vi "ECGfirst.vi"() -> ()   [LabVIEW 2015]
uses:
  <vilib>/Instr/_visa.llb/VISA Configure Serial Port (Instr).vi
panel:
  in  "Stop Button 2":bool
  in  "Menus":enum32{"Configuración", "Variables", "Graficas"}(tab)
  out "A case":u16
  in  "Text & Pict Ring 2":u16(ring) items=["Tiempo Real"=1, "Desconectado"=2, "Datos almaceados"=3, "Alarma Medir"=0]
  in  "LECTURA":bool
  in  "ESCRITURA":bool
  in  "VISA resource name":refnum<visa-resource-name>
  out "Al PIC":string
  out "Array 2":dbl[](array[numeric])
  out "read buffer":string
  out "Table":string[][](table)
  in  "Open Button":bool
  out "Table Control":string[][](table)
  in  "path":path
  out "Waveform Chart":dbl(graph)
  # "ELECTROCARDIOGRAFO \nPORTATIL"
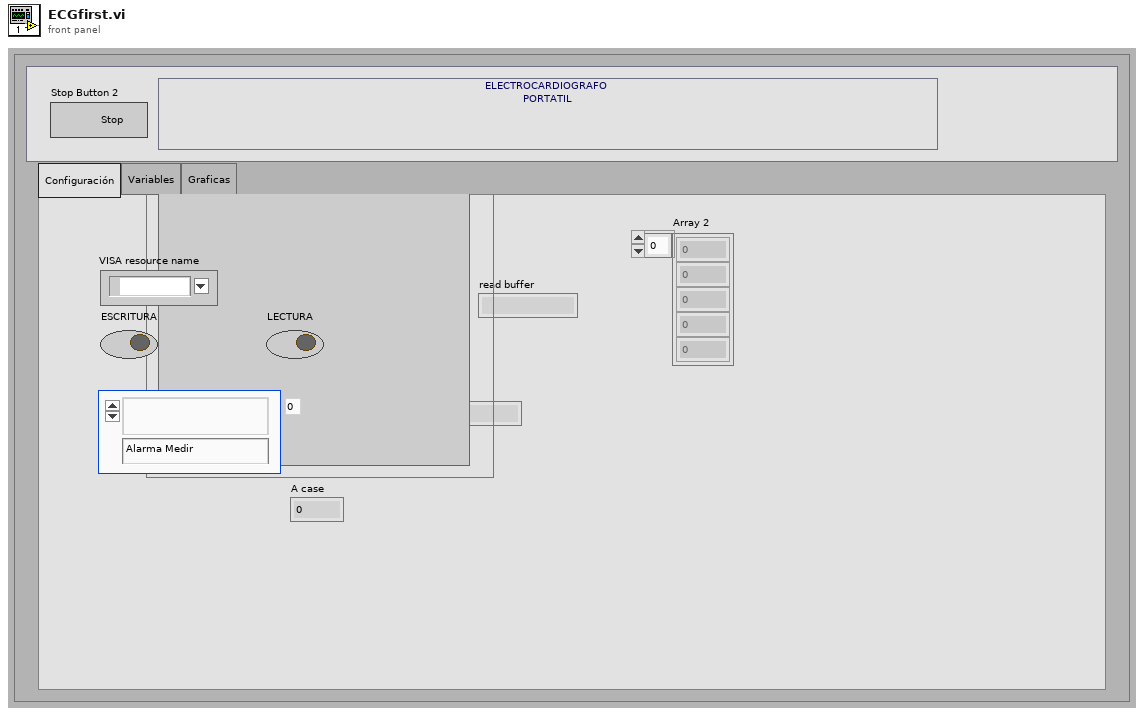
[diagram p1: front panel]
types:
  T1 = cluster{"Excel._Application":refnum<k7>, "Workbooks":refnum<k7>}
  T2 = cluster{"Excel._Application":refnum<k7>, "Workbooks":refnum<k7>, "Open":refnum<k7>}
  T3 = cluster{"Excel._Application":refnum<k7>, "Workbooks":refnum<k7>, "Open":refnum<k7>, "Worksheets":refnum<k7>, "Excel._Worksheet":refnum<k7>}
  T4 = cluster{"unsigned byte array[0]":u8, "unsigned byte array[1]":u8, "unsigned byte array[2]":u8, "unsigned byte array[3]":u8, "unsigned byte array[4]":u8, "unsigned byte array[5]":u8, "unsigned byte array[6]":u8, "unsigned byte array[7]":u8, "unsigned byte array[8]":u8}
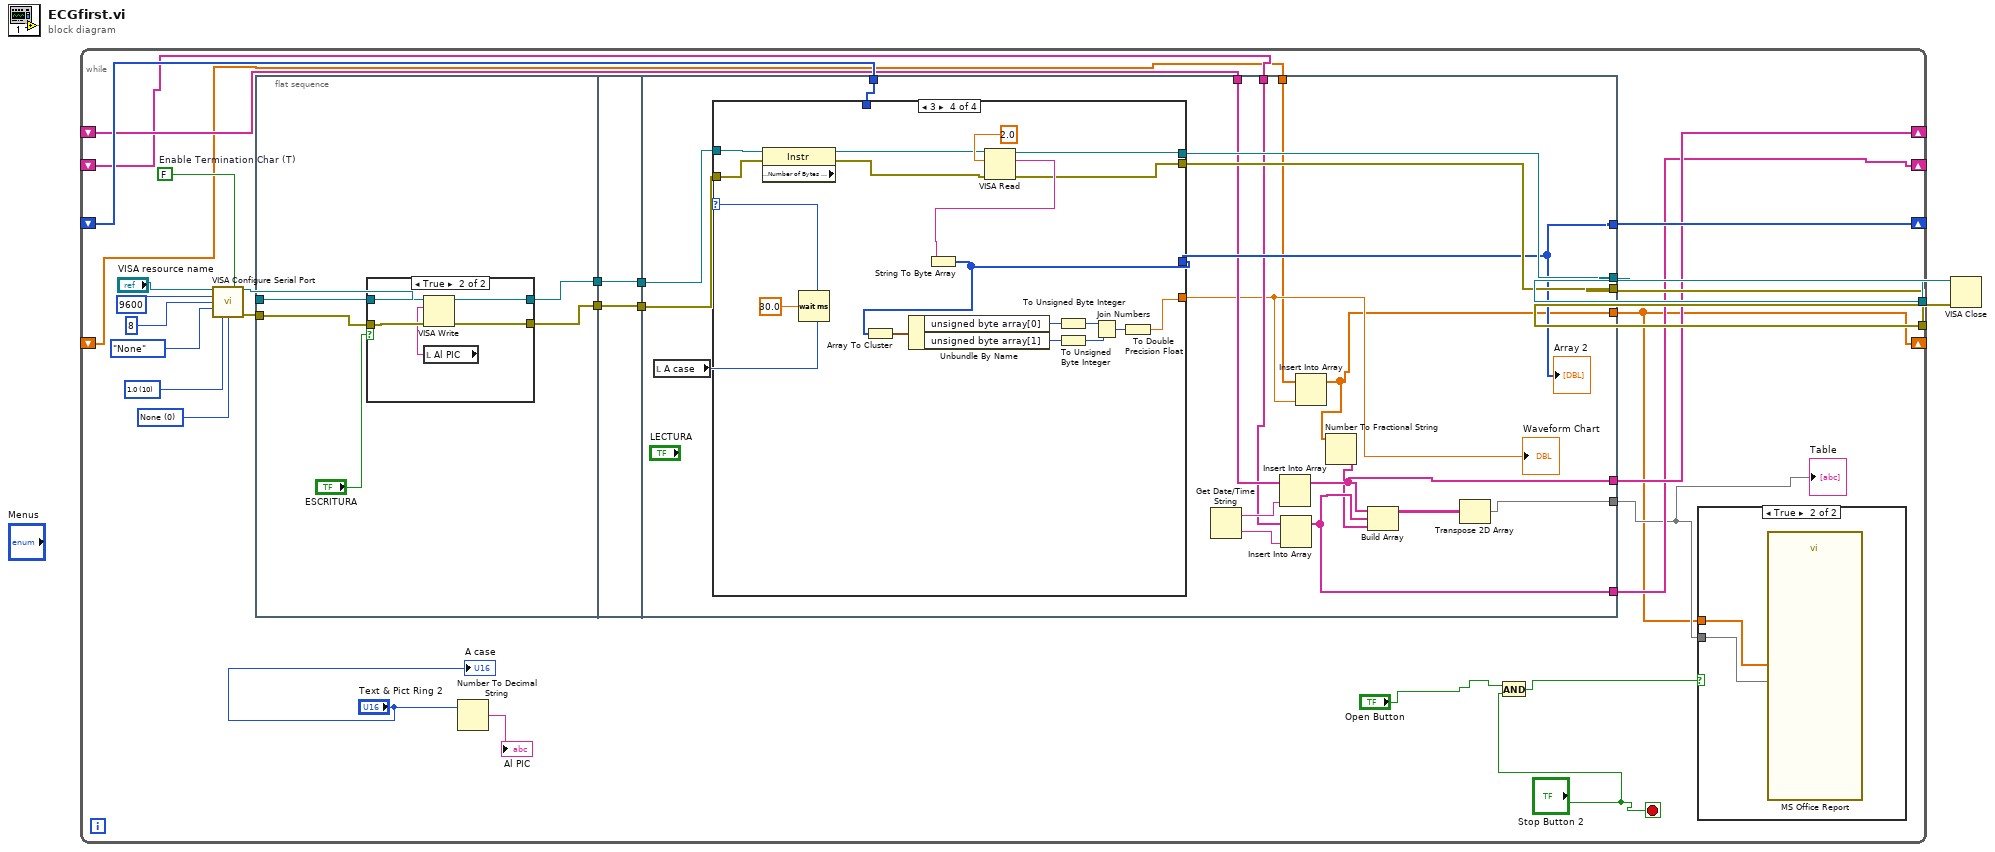
[diagram p0: block diagram]
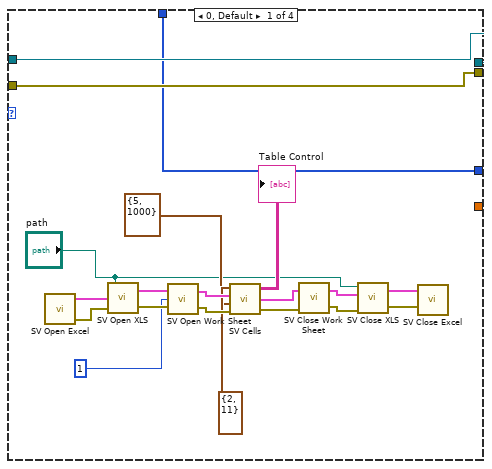
[diagram p4: hidden frame]
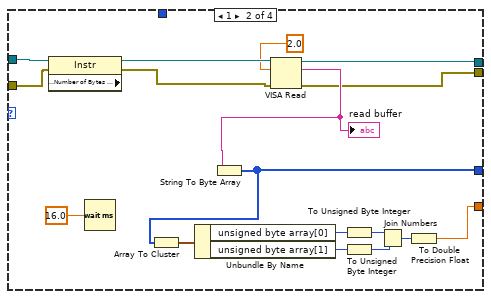
[diagram p5: hidden frame]
diagram:
  n1 = while {
    tunnel: [w17] -> w2
    tunnel: [w15] -> w1
    shift-right: [w14] -> _
    shift-left: _ -> [w13]
    shift-right: [w12] -> _
    shift-left: _ -> [w11]
    shift-right: [w10] -> _
    shift-left: _ -> [w9]
    shift-right: [w3] -> _
    shift-left: _ -> [w4]
    stop <- "Stop Button 2" stop-if-true
    w31 = u16 0 items=["None", "XON/XOFF", "RTS/CTS", "XON/XOFF & RTS/CTS", "DTR/DSR", "XON/XOFF & DTR/DSR"] ("flow control (0:none)")
    w30 = FALSE  # Enable Termination Char (T)
    w27 = u16 10 items=["1.0"=10, "1.5"=15, "2.0"=20] ("stop bits (10: 1 bit)")
    n2 = call-poly "VISA Configure Serial Port"("VISA resource name"="VISA resource name", "Enable Termination\nChar (T)"=w30, "baud rate (9600)"=9600 ("Numeric 2"), "data bits (8)"=u16 8, "parity (0:none)"=enum16{"None", "Odd", "Even", "Mark", "Space"}."None", "stop bits (10: 1 bit)"=w27, "flow control (0:none)"=w31) -> ("VISA resource name out"=w19:refnum<visa-resource-name>, "error out"=w18:errorcluster)  [unwired: 7 in]
    n3 = flat-sequence {
      tunnel: [w35] -> w23
      tunnel: [w34] -> w22
      tunnel: w19 -> [w38]
      tunnel: w18 -> [w37]
      tunnel: [w47] -> w21
      tunnel: w23 -> [w47]
      tunnel: w22 -> [w46]
      tunnel: [w46] -> w20
      tunnel: w21 -> [w65]
      tunnel: w20 -> [w64]
      tunnel: [w63] -> w17
      tunnel: [w62] -> w15
      tunnel: [w61] -> w14
      tunnel: w13 -> [w60]
      tunnel: [w57] -> w12
      tunnel: w11 -> [w56]
      tunnel: [w55] -> w10
      tunnel: w9 -> [w54]
      tunnel: [w52] -> w8
      tunnel: [w48] -> w3
      tunnel: w4 -> [w50]
      frame #0 {
        n4 = case shown="True" "ESCRITURA" {
          tunnel: w38 -> [w40 w45]
          tunnel: [w40 w41] -> w35
          tunnel: [w39 w44] -> w34
          tunnel: w37 -> [w39 w43]
          frame False {
          }
          frame True {
            n5 = local read "Al PIC"() -> (w42:string)
            n6 = VISA Write(VISA resource name=w45, write buffer=w42, error in (no error)=w43) -> (VISA resource name out=w41:refnum<visa-resource-name>, error out=w44:errorcluster)  [unwired: 1 out]
          }
        }
      }
      frame #1 {
      }
      frame #2 {
        n7 = local read "A case"() -> (w66:u16)
        n8 = case shown="3" w66 {
          tunnel: w65 -> [w86 w92 w106 w112]
          tunnel: w64 -> [w85 w91 w105 w111]
          tunnel: [w86 w90 w106 w110] -> w63
          tunnel: [w85 w89 w105 w109] -> w62
          tunnel: [_ w88 _ w107] -> w51
          tunnel: [w84 w87 w104 w108] -> w61
          tunnel: w60 -> [w84 _ w104 _]
          frame 0, Default {
            n9 = call "SV Open Excel.vi"() -> ("error out"=w83:errorcluster, "Refnum Cluster"=w82:T1)  [unwired: 1 in]
            n10 = call "SV Open XLS.vi"("error in"=w83, "Refnum Cluster In"=w82, "path"="path") -> ("error out"=w80:errorcluster, "Refnum Cluster Out"=w81:T2)
            n11 = call "SV Open Work Sheet.vi"("error in (no error)"=w80, "Sheet"=1, "Refnum Cluster In"=w81) -> ("error out"=w78:errorcluster, "Refnum Cluster Out"=w79:T3)
            n12 = call "SV Cells.vi"("error in"=w78, "End 2"=cluster{"Column":i32, "Row":i32} {"Column"=5, "Row"=1000}, "Refnum Cluster In"=w79, "Start 2"=cluster{"Column":i32, "Row":i32} {"Column"=2, "Row"=11}) -> ("Error Out"=w77:errorcluster, "Refnum Cluster Out"=w76:T3, "Data"=→"Table Control":string[][])
            n13 = call "SV Close Work Sheet.vi"("error in (no error)"=w77, "Refnum Cluster In"=w76) -> ("error out"=w74:errorcluster, "Refnum Cluster Out"=w75:T2)
            n14 = call "SV Close XLS.vi"("error in (no error)"=w74, "Refnum Cluster In"=w75, "path 2"="path") -> ("error out"=w72:errorcluster, "Refnum Cluster Out"=w73:T1)  [unwired: 1 in]
            n15 = call "SV Close Excel.vi"("error in (no error)"=w72, "Refnum Cluster In"=w73) -> ()  [unwired: 1 out]
          }
          frame 1 {
            n16 = property class="Instr" props=["Serial Settings:Number of Bytes at Serial Port"](reference=w92, error in=w91) -> (reference out=w101:refnum<visa-resource-name>, error out=w102:errorcluster)  [unwired: 1 out]
            n17 = Wait (ms)(milliseconds to wait=sgl 16.0 ("Vielfache von ms")) -> ()  [unwired: 1 out]
            n18 = VISA Read(VISA resource name=w101, byte count=2.0 ("BYTES A LEER"), error in (no error)=w102) -> (VISA resource name out=w90:refnum<visa-resource-name>, read buffer=w93:string, error out=w89:errorcluster)  [unwired: 1 out]
            "read buffer" <- w93
            n19 = String To Byte Array(string=w93) -> (unsigned byte array=w87:u8[])
            n20 = Array To Cluster(array=w87) -> (cluster=w94:T4)
            n21 = Unbundle By Name(w94) -> ("unsigned byte array[0]"=w98:u8, "unsigned byte array[1]"=w99:u8)
            n22 = To Unsigned Byte Integer(number=w98) -> (unsigned 8bit integer=w95:u8)
            n23 = To Unsigned Byte Integer(number=w99) -> (unsigned 8bit integer=w96:u8)
            n24 = Join Numbers(hi=w95, lo=w96) -> ((hi.lo)=w97:u16)
            n25 = To Double Precision Float(number=w97) -> (double precision float=w88:dbl)
          }
          frame 2 {
          }
          frame 3 {
            n26 = property class="Instr" props=["Serial Settings:Number of Bytes at Serial Port"](reference=w112, error in=w111) -> (reference out=w115:refnum<visa-resource-name>, error out=w114:errorcluster)  [unwired: 1 out]
            n27 = Wait (ms)(milliseconds to wait=sgl 30.0 ("Vielfache von ms")) -> ()  [unwired: 1 out]
            n28 = VISA Read(VISA resource name=w115, byte count=2.0 ("BYTES A LEER"), error in (no error)=w114) -> (VISA resource name out=w110:refnum<visa-resource-name>, read buffer=w123:string, error out=w109:errorcluster)  [unwired: 1 out]
            n29 = String To Byte Array(string=w123) -> (unsigned byte array=w108:u8[])
            n30 = Array To Cluster(array=w108) -> (cluster=w122:T4)
            n31 = Unbundle By Name(w122) -> ("unsigned byte array[0]"=w118:u8, "unsigned byte array[1]"=w117:u8)
            n32 = To Unsigned Byte Integer(number=w118) -> (unsigned 8bit integer=w121:u8)
            n33 = To Unsigned Byte Integer(number=w117) -> (unsigned 8bit integer=w120:u8)
            n34 = Join Numbers(hi=w121, lo=w120) -> ((hi.lo)=w119:u16)
            n35 = To Double Precision Float(number=w119) -> (double precision float=w107:dbl)
          }
        }
        "Waveform Chart" <- w51
        "Array 2" <- w61
        n36 = Get Date/Time String() -> (date string=w59:string, time string=w58:string)  [unwired: 3 in]
        n37 = Insert Into Array(array=w56, new element=w59) -> (w57:string[])  [unwired: 1 in]
        n38 = Insert Into Array(array=w54, new element=w58) -> (w55:string[])  [unwired: 1 in]
        n39 = Insert Into Array(array=w50, new element=w51) -> (w48:dbl[])  [unwired: 1 in]
        n40 = Number To Fractional String(number=w48) -> (F-format string=w49:string[])  [unwired: 3 in]
        n41 = Build Array(w57, w55, w49) -> (w53:string[][])
        n42 = Transpose 2D Array(2D array=w53) -> (transposed array=w52:string[][])
      }
    }
    n43 = Number To Decimal String(number="Text & Pict Ring 2") -> (decimal integer string=→"Al PIC":string)  [unwired: 1 in]
    n44 = And(x="Open Button", y="Stop Button 2") -> (x .and. y?=w5:bool)
    n45 = case shown="True" w5 {
      tunnel: w3 -> [_ w33]
      tunnel: w8 -> [_ w32]
      frame False {
      }
      frame True {
        n46 = call "MS Office Report"("chart"=w33, "data"=w32) -> ()  [unwired: 25 in, 1 out]
      }
    }
    "A case" <- "Text & Pict Ring 2"
    "Table" <- w8
  }
  n47 = VISA Close(VISA resource name=w2, error in (no error)=w1) -> ()  [unwired: 1 out]
